vi "ENPH354_7SegOutput(SubVI).vi"(11 "Knob":dbl) -> (3 "Array":bool[](array[boolean]))   [LabVIEW 2020]
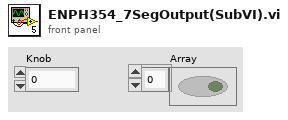
[diagram p1: front panel]
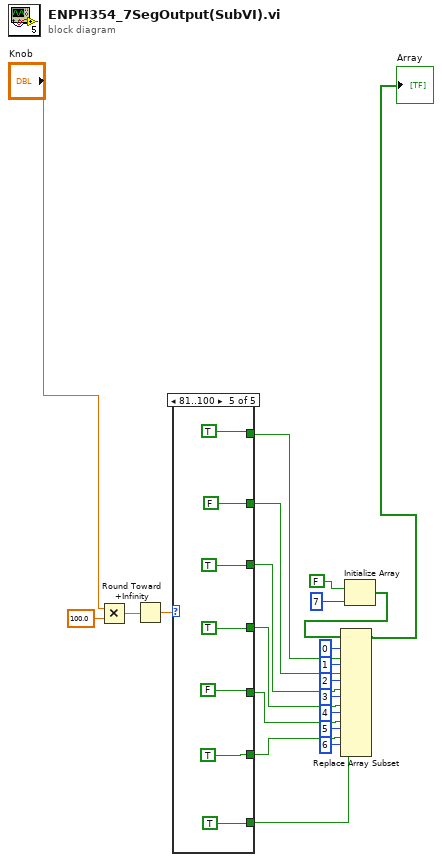
[diagram p0: block diagram]
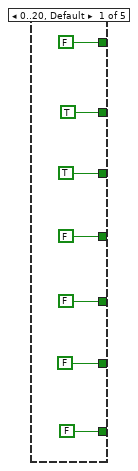
[diagram p2: hidden frame]
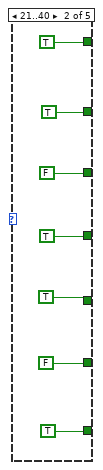
[diagram p3: hidden frame]
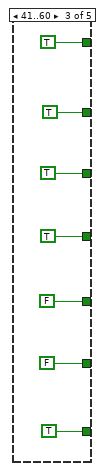
[diagram p4: hidden frame]
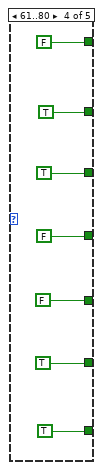
[diagram p5: hidden frame]
diagram:
  n1 = Multiply(x="Knob", y=100.0) -> (x*y=w20:dbl)
  n2 = Round Toward +Infinity(x=w20) -> (ceil(x): smallest int >= x=w19:dbl)
  n3 = case shown="81..100" w19 {
    tunnel: [FALSE TRUE TRUE FALSE TRUE] -> w15
    tunnel: [TRUE TRUE TRUE TRUE FALSE] -> w14
    tunnel: [TRUE FALSE TRUE TRUE TRUE] -> w10
    tunnel: [FALSE TRUE TRUE FALSE TRUE] -> w8
    tunnel: [FALSE TRUE FALSE FALSE FALSE] -> w6
    tunnel: [FALSE FALSE FALSE TRUE TRUE] -> w2
    tunnel: [FALSE TRUE TRUE TRUE TRUE] -> w3
    frame 0..20, Default {
    }
    frame 21..40 {
    }
    frame 41..60 {
    }
    frame 61..80 {
    }
    frame 81..100 {
    }
  }
  n4 = Initialize Array(FALSE, 7 ("dimension size")) -> (w16:bool[])
  n5 = Replace Array Subset(array=w16, new element #1=w15, index #1=0 ("index"), new element #2=w14, index #2=1 ("index"), new element #3=w10, index #3=2 ("index"), new element #4=w8, index #4=3 ("index"), new element #5=w6, index #5=4 ("index"), new element #6=w2, index #6=5 ("index"), new element #7=w3, index #7=6 ("index")) -> (→"Array":bool[])
